vi "Kelompok 3_Tipe Data.vi"() -> ()   [LabVIEW 2020]
panel:
  out "Numeric 6":i32
  in  "Numeric 5":i32
  out "String 4":string
  in  "String 3":string
  out "output cluster":cluster{"Nama":string, "Umur":i32, "L/P":bool}
  in  "L/P":bool
  in  "Umur":i32
  in  "Nama":string
  out "appended array":dbl[](array[numeric])
  in  "element 4":dbl
  in  "element 3":dbl
  in  "element 2":dbl
  in  "element":dbl
  out "Boolean 2":bool
  in  "Boolean":bool
  out "Numeric 4":i32
  in  "Numeric 3":i32
  out "Numeric 2":dbl
  in  "Numeric":dbl
  out "String 2":string
  in  "String":string
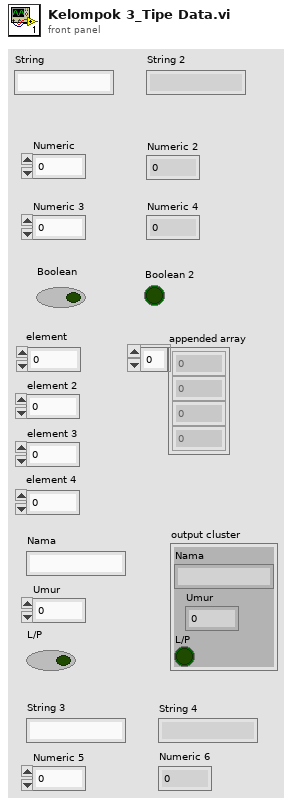
[diagram p1: front panel]
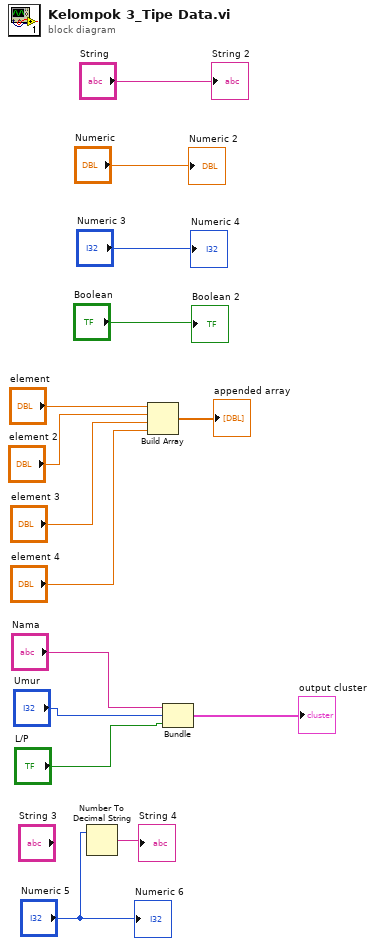
[diagram p0: block diagram]
diagram:
  n1 = Number To Decimal String(number="Numeric 5") -> (decimal integer string=→"String 4":string)  [unwired: 1 in]
  n2 = Build Array("element", "element 2", "element 3", "element 4") -> (→"appended array":dbl[])
  n3 = Bundle("Nama"="Nama", "Umur"="Umur", "L/P"="L/P") -> (→"output cluster":cluster{"Nama":string, "Umur":i32, "L/P":bool})  [unwired: 1 in]
  "String 2" <- "String"
  "Numeric 2" <- "Numeric"
  "Numeric 4" <- "Numeric 3"
  "Boolean 2" <- "Boolean"
  "Numeric 6" <- "Numeric 5"
